vi "Open Report File.vi"(8 "error in (no error)":errorcluster, 11 "Report In":refnum<class "Report.lvclass">) -> (0 "error out":errorcluster, 3 "Report Out":refnum<class "Report.lvclass">)   [LabVIEW 2020, in "Report Generation.lvlib" / "Report.lvclass"]
uses:
  Report.lvclass
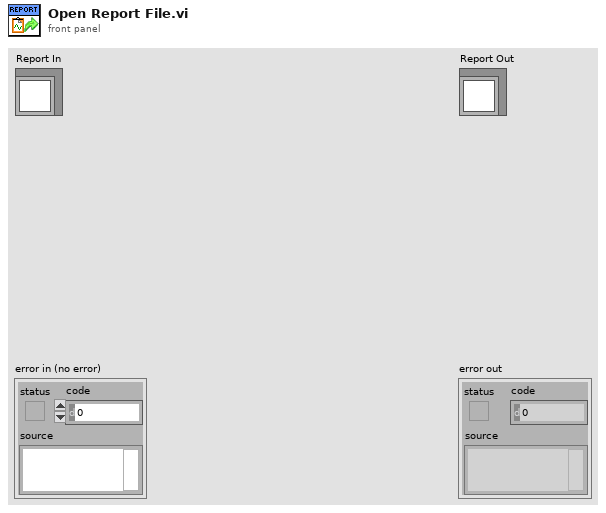
[diagram p1: front panel]
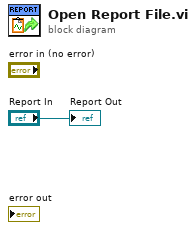
[diagram p0: block diagram]
diagram:
  "Report Out" <- "Report In"
